vi "Decoder.vi"(2 "Data frame":u16[](array[numeric])) -> (8 "Pot 1":u16, 9 "Pot 2":u16, 10 "SW1 H":bool, 12 "SW1 L":bool, 14 "SW2 H":bool, 15 "SW2 L":bool, 16 "SW3 H":bool, 17 "SW3 L":bool, 18 "SW4 H":bool, 19 "SW4 L":bool)   [LabVIEW 2016]
panel:
  out "QUE?":bool
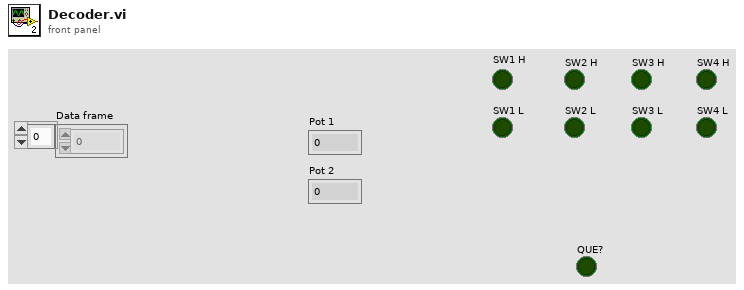
[diagram p1: front panel]
types:
  T1 = cluster{"Data frame[0]":u16, "Data frame[1]":u16, "Data frame[2]":u16, "Data frame[3]":u16, "Data frame[4]":u16, "Data frame[5]":u16, "Data frame[6]":u16, "Data frame[7]":u16, "Data frame[8]":u16}
  T2 = cluster{"Boolean array[0]":bool, "Boolean array[1]":bool, "Boolean array[2]":bool, "Boolean array[3]":bool, "Boolean array[4]":bool, "Boolean array[5]":bool, "Boolean array[6]":bool, "Boolean array[7]":bool, "Boolean array[8]":bool}
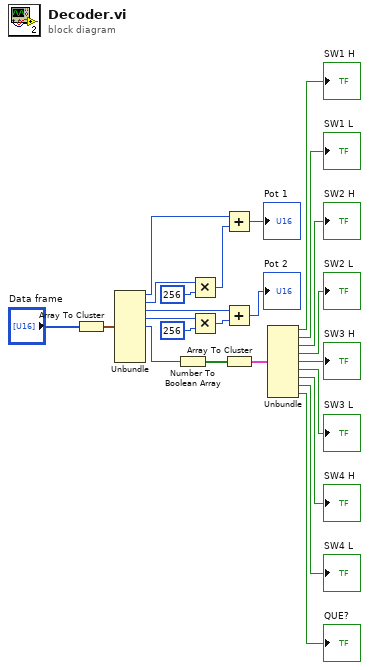
[diagram p0: block diagram]
diagram:
  n1 = Array To Cluster(array="Data frame") -> (cluster=w23:T1)
  n2 = Unbundle(w23) -> ("Data frame[0]"=w22:u16, "Data frame[1]"=w21:u16, "Data frame[2]"=w14:u16, "Data frame[3]"=w13:u16, "Data frame[4]"=w12:u16)  [unwired: 4 out]
  n3 = Number To Boolean Array(number=w12) -> (Boolean array=w11:bool[])
  n4 = Multiply(x=w21, y=u16 256) -> (x*y=w19:u16)
  n5 = Multiply(x=w13, y=u16 256) -> (x*y=w16:u16)
  n6 = Add(x=w22, y=w19) -> (x+y=→"Pot 1":u16)
  n7 = Add(x=w14, y=w16) -> (x+y=→"Pot 2":u16)
  n8 = Array To Cluster(array=w11) -> (cluster=w10:T2)
  n9 = Unbundle(w10) -> ("Boolean array[0]"=→"SW1 H":bool, "Boolean array[1]"=→"SW1 L":bool, "Boolean array[2]"=→"SW2 H":bool, "Boolean array[3]"=→"SW2 L":bool, "Boolean array[4]"=→"SW3 H":bool, "Boolean array[5]"=→"SW3 L":bool, "Boolean array[6]"=→"SW4 H":bool, "Boolean array[7]"=→"SW4 L":bool, "Boolean array[8]"=→"QUE?":bool)
